vi "heating_reg.vi"(0 "SP":dbl caption="setpoint" step=0.01 format="%.2f", 1 "Y":T3={"Y_HSw"=1, "Y_HSetState"=enum."auto", "Y_ASetState"=enum."auto", "Y_DSetState"=enum."auto"}, 2 "Z":cluster{"Z_State":T6, "ZM_State":T7}={"Z_State"=enum."alarm", "ZM_State"=enum."initialization"}, 3 "XB24 (F)":bool, 5 "PV":dbl step=0.01 format="%.2f", 7 "Y_H":dbl step=1.0, 9 "controls Y":cluster{"Y_L":dbl, "Y_A":dbl, "Y_D":dbl} {"Y_D" format="%#_13g"; "Y_A" format="%#_13g"; "Y_L" format="%.2f"}, 12 "REG param":T8={"proportional gain (Kc)"=1.0, "integral time (Ti, s)"=10.0, "derivative time (Td, s)"=1.0, "output high"=100.0, "output high start"=40.0, "output high stop"=40.0, "alr value"=0.0, "output low"=0.0, "output rate (EGU/s)"=5.0, "setpoint max"=100.0, "setpoint rate (EGU/min)"=10.0, "stop rate (EGU/min)"=5.0} {"setpoint max" format="%.2f"; "stop rate (EGU/min)" min=0.001 format="%.2f"; "setpoint rate (EGU/min)" min=0.001 format="%.2f"; "output high stop" format="%.2f"; "output high start" format="%.2f"; "output rate (EGU/s)" min=0.001 format="%.2f"; "output low" format="%.2f"; "alr value" format="%.2f"; "output high" format="%.2f"; "derivative time (Td, s)" format="%.3f"; "integral time (Ti, s)" format="%.3f"; "proportional gain (Kc)" format="%.3f"}, 13 "PV_State":T1) -> (4 "Y_State":T4={"Y_Source"=enum."local disabled", "Y_SetState"=enum."auto", "SP_Set"=0.0, "SP"=0.0, "PV"=0.0, "Y"=0.0, "Y_State"={"code"=0, "visible"=FALSE, "color"=0}, "YB"=FALSE} {"SP" step=0.01 format="%.2f"; "Y" format="%.2f"; "PV" step=0.01 format="%.2f"; "SP_Set" step=0.01 format="%.2f"}, 6 "Y":dbl format="%.2f", 8 "T":u32, 10 "End":bool, 14 "YB":bool)   [LabVIEW 2019, in "Heating.lvlib"]
uses:
  Heating.lvlib
  ctl/Z_State.ctl
  ctl/ZM_State.ctl
  ctl/Y_short.ctl
  ctl/Y_source.ctl
  ctl/Y_state.ctl
  Inputs/Ctl/Parameter State short.ctl
  Reg/PID Output Rate Limiter Ext.vi
  Reg/PID Timing Estimation Ext.vi
  Reg/PID Output Rate Limiter.vi
  Logik/fronts.vi
  Reg/PID Timing Estimation.vi
  Reg/control.lvlib
  Userlib.lvlib
  Inputs/Inputs.lvlib
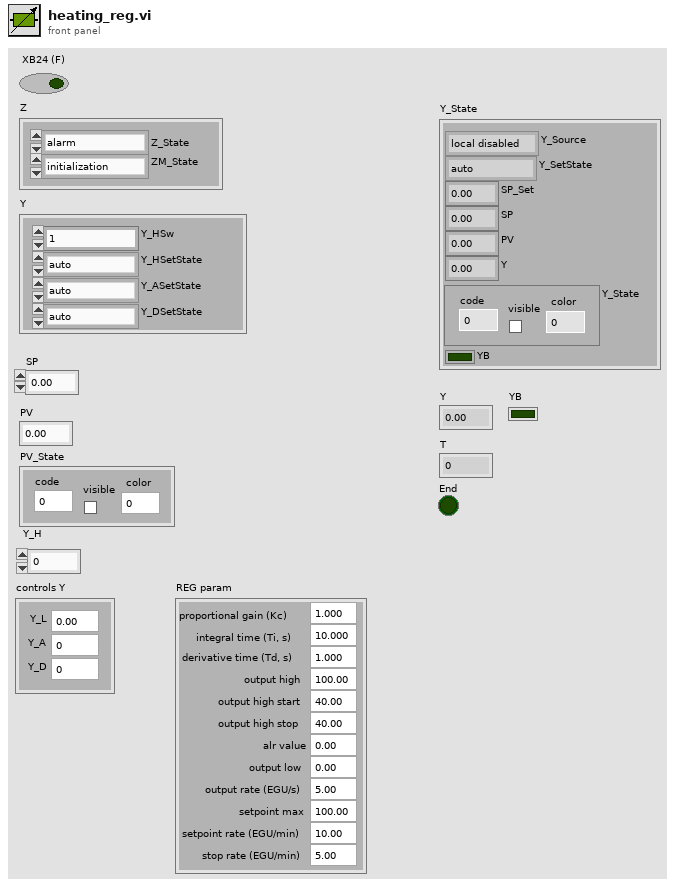
[diagram p1: front panel]
types:
  T1 = typedef "Inputs.lvlib/Parameter State short.ctl" = cluster{"code":i32, "visible":bool, "color":u32}
  T2 = typedef "Heating.lvlib/Y_state.ctl" = enum8{"initialize", "alarm", "min", "stop", "hand", "auto", "max"}
  T3 = cluster{"Y_HSw":u32, "Y_HSetState":T2, "Y_ASetState":T2, "Y_DSetState":T2}
  T4 = typedef "Heating.lvlib/Y_short.ctl" = cluster{"Y_Source":T5, "Y_SetState":T2, "SP_Set":dbl, "SP":dbl, "PV":dbl, "Y":dbl, "Y_State":T1, "YB":bool}
  T5 = typedef "Heating.lvlib/Y_source.ctl" = enum8{"initialize", "local disabled", "local hand", "hand", "auto", "dist"}
  T6 = typedef "Heating.lvlib/Z_State.ctl" = enum8{"initialization", "alarm", "disabled", "not ready", "stop ready", "reserv", "switched off", "reserv2", "switched on", "check", "on min", "decrease out", "on", "increase out", "on max"}
  T7 = typedef "Heating.lvlib/ZM_State.ctl" = enum8{"initialization", "stop", "start_cmd", "contactor_on_cmd", "heating", "on", "stop_cmd", "power_down", "contactor_off_cmd", "cooling", "restart_delay"}
  T8 = cluster{"proportional gain (Kc)":dbl, "integral time (Ti, s)":dbl, "derivative time (Td, s)":dbl, "output high":dbl, "output high start":dbl, "output high stop":dbl, "alr value":dbl, "output low":dbl, "output rate (EGU/s)":dbl, "setpoint max":dbl, "setpoint rate (EGU/min)":dbl, "stop rate (EGU/min)":dbl}
  T9 = typedef "control.lvlib/PID param.ctl" = cluster{"proportional gain (Kc)":dbl, "integral time (Ti, s)":dbl, "derivative time (Td, s)":dbl, "output high":dbl, "alr value":dbl, "output low":dbl, "output rate (EGU/s)":dbl, "dt (s)":dbl}
  T10 = enum8{"alarm", "min", "stop", "hand", "auto", "max"}
  T11 = cluster{"Y_Source":T5, "Y_SetState":T2, "SP":dbl, "output":dbl, "PV":dbl, "set output":dbl, "PV_State":T1, "Y":bool}
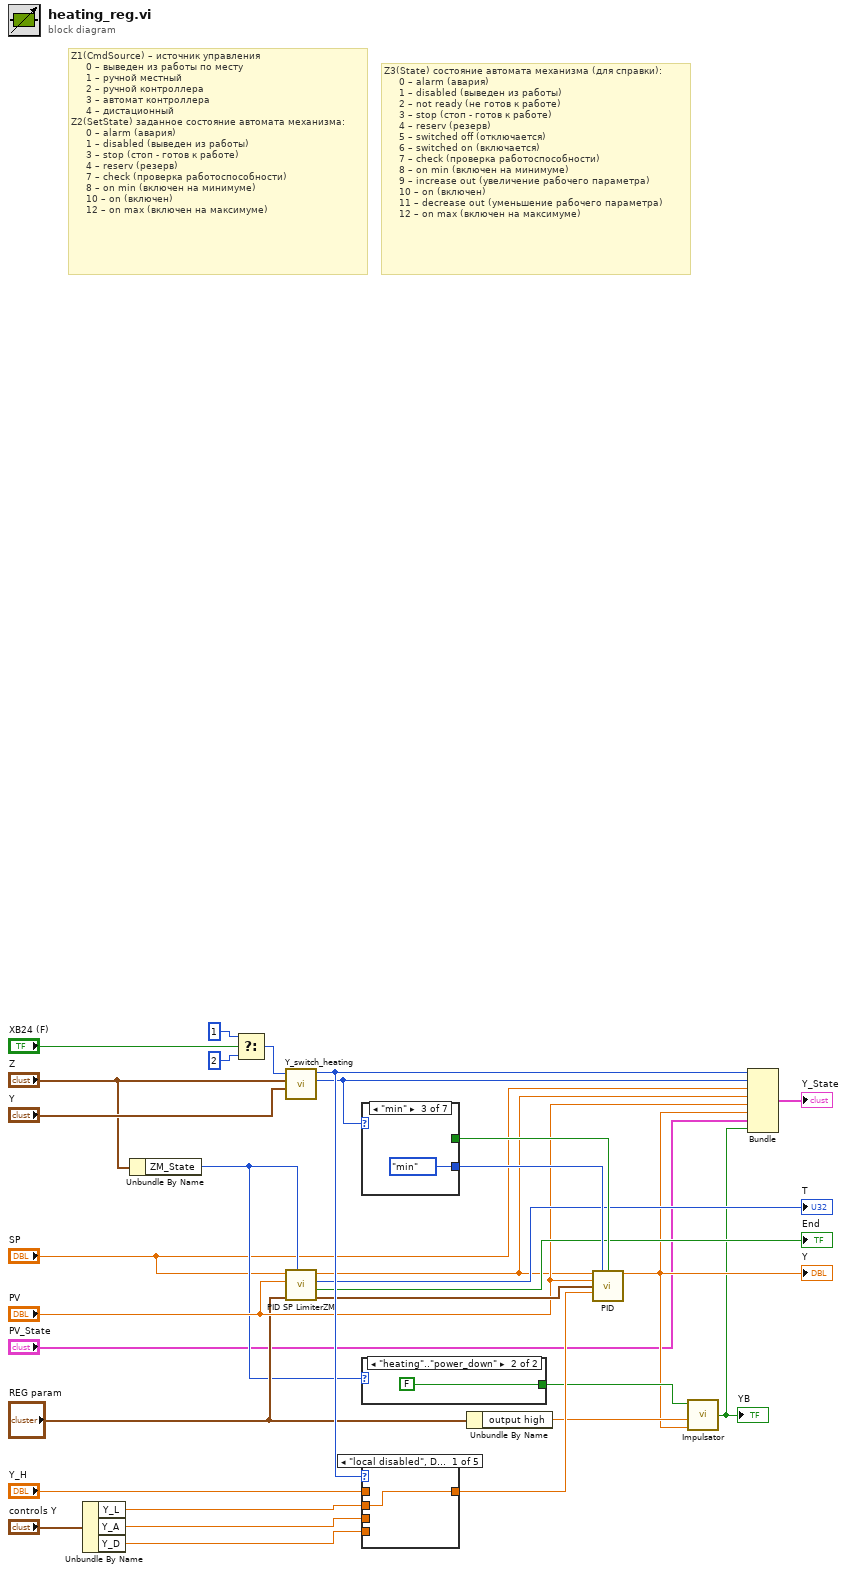
[diagram p0: block diagram]
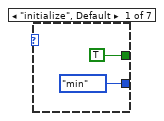
[diagram p2: hidden frame]
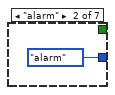
[diagram p3: hidden frame]
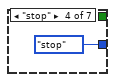
[diagram p4: hidden frame]
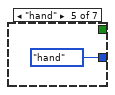
[diagram p5: hidden frame]
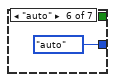
[diagram p6: hidden frame]
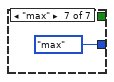
[diagram p7: hidden frame]
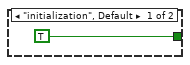
[diagram p8: hidden frame]
diagram:
  # "Z1(CmdSource) – источник управления\n     0 – выведен из работы по месту\n     1 – ручной местный\n     2 – ручной контроллера\n     3 – автомат контроллера\n     4 – дистационный\nZ2(SetState) заданное состояние автомата механизма:\n     0 – alarm (авария)\n     1 – disabled (выведен из работы)\n     3 – stop (стоп - готов к работе)\n     4 – reserv (резерв)\n     7 – check (проверка работоспособности)\n     8 – on min (включен на минимуме)\n     10 – on (включен)\n     12 – on max (включен на максимуме)"
  # "Z3(State) состояние автомата механизма (для справки):\n     0 – alarm (авария)\n     1 – disabled (выведен из работы)\n     2 – not ready (не готов к работе)\n     3 – stop (стоп - готов к работе)\n     4 – reserv (резерв)\n     5 – switched off (отключается)\n     6 – switched on (включается)\n     7 – check (проверка работоспособности)\n     8 – on min (включен на минимуме)\n     9 – increase out (увеличение рабочего параметра)\n     10 – on (включен)\n     11 – decrease out (уменьшение рабочего параметра)\n     12 – on max (включен на максимуме)"
  n1 = Unbundle By Name("controls Y") -> ("Y_L"=w28:dbl, "Y_A"=w29:dbl, "Y_D"=w27:dbl)
  n2 = Unbundle By Name("Z") -> ("ZM_State"=w6:T7)
  n3 = Select(t=u32 1, s="XB24 (F)", f=u32 2 ("Y_HSw")) -> (s? t:f=w22:u32)
  n4 = call "Y_switch_heating.vi"("Y"="Y", "Z"="Z", "Y_LSw (2-auto)"=w22) -> ("Y_SetState"=w18:T2, "Y_Source"=w20:T5)  [unwired: 7 in]
  n5 = call "PID SP LimiterZM.vi"("ZM_State"=w6, "REG param"="REG param", "PV"="PV", "SP"="SP") -> ("PID param"=w15:T9, "End"=→"End":bool, "T"=→"T":u32, "output"=w5:dbl)  [unwired: 4 in]
  n6 = case shown="\"min\"" w18 {
    tunnel: [T10."min" ("X1(SetState)") T10."alarm" ("X1(SetState)") T10."min" ("X1(SetState)") T10."stop" ("X1(SetState)") T10."hand" ("X1(SetState)") T10."auto" ("X1(SetState)") T10."max" ("X1(SetState)")] -> w17
    tunnel: [TRUE _ _ _ _ _ _] -> w16
    frame "initialize", Default {
    }
    frame "alarm" {
    }
    frame "min" {
    }
    frame "stop" {
    }
    frame "hand" {
    }
    frame "auto" {
    }
    frame "max" {
    }
  }
  n7 = case shown="\"heating\"..\"power_down\"" w6 {
    tunnel: [TRUE FALSE] -> w8
    frame "initialization", Default {
    }
    frame "heating".."power_down" {
    }
  }
  n8 = case shown="\"local disabled\", Default" w20 {
    tunnel: "Y_H" -> [_ _ w43 _ _]
    tunnel: w28 -> [w41 w42 _ _ _]
    tunnel: w27 -> [_ _ _ _ w45]
    tunnel: [w41 w42 w43 w44 w45] -> w25
    tunnel: w29 -> [_ _ _ w44 _]
    frame "local disabled", Default {
    }
    frame "local hand" {
    }
    frame "hand" {
    }
    frame "auto" {
    }
    frame "dist" {
    }
  }
  n9 = Unbundle By Name("REG param") -> ("output high"=w10:dbl)
  n10 = call "PID.vi"("setpoint"=w5, "X1(SetState)"=w17, "reinitialize? (F)"=w16, "process variable"="PV", "PID param"=w15, "manual control"=w25) -> ("set output"=w7:dbl)  [unwired: 7 in, 2 out]
  "Y" <- w7
  n11 = call "Impulsator.vi"("PV"=w7, "upper limit"=w10, "Initialise"=w8) -> ("Y"=w3:bool)  [unwired: 1 in]
  "YB" <- w3
  n12 = Bundle("Y_Source"=w20, "Y_SetState"=w18, "SP"="SP", "output"=w5, "PV"="PV", "set output"=w7, "PV_State"="PV_State", "Y"=w3) -> (→"Y_State":T11)  [unwired: 1 in]
